vi "Cam.vi"() -> ()   [LabVIEW 2021]
uses:
  <vilib>/userdefined/High Color/IMAQdx.ctl
  <vilib>/MakerHub/LINX/Public/Peripherals/Digital/Digital Write 1 Chan.vi
  <vilib>/MakerHub/LINX/Public/Peripherals/Digital/Digital Write N Chans.vi
  <vilib>/MakerHub/LINX/Private/Local IO/LinxDigitalWrite.vi
  <vilib>/MakerHub/LINX/Public/Utilities/Check Channel.vi
  <vilib>/MakerHub/LINX/Public/Utilities/Open Serial.vi
  <vilib>/MakerHub/LINX/Private/Utilties/Generate Error.vi
  <vilib>/vision/driver/NI_Vision_Acquisition_Software.lvlib
  <vilib>/vision/NI_Vision_Development_Module.lvlib
  <vilib>/MakerHub/LINX/LMH-LINX.lvlib
panel:
  out "Loop Rate (Hz)":u32
  in  "Digital Output Channel":u8=13
  in  "Serial Port":refnum<visa-resource-name>
  out "EJE Y":sgl
  out "EJE X":sgl
  in  "Reconocer":bool
  out "Muestra":T1(plugin-control)
  out "Imagen":T1(plugin-control)
  in  "Camara":T2
  in  "stop":bool
  # "ELECTROMARK VISION ARTIFICIAL"
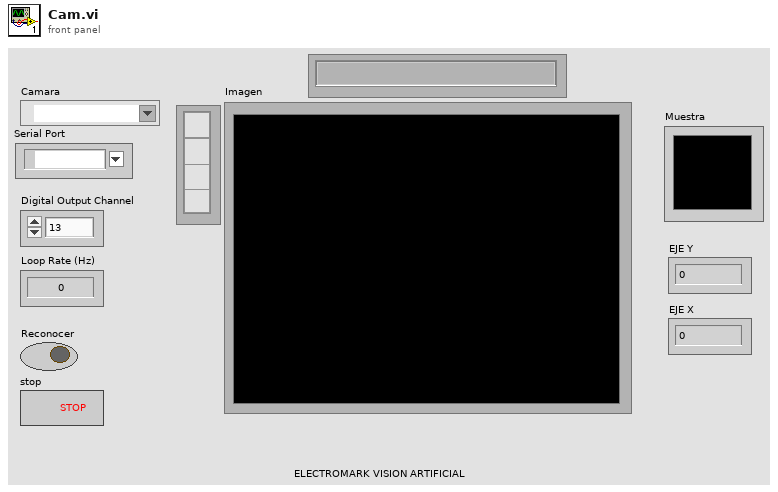
[diagram p1: front panel]
types:
  T1 = typedef "IMAQ Image.ctl" = refnum<image>
  T2 = typedef "IMAQdx.ctl" = refnum<k21>
  T3 = typedef "Image Type" = u32
  T4 = typedef "LMH-LINX.lvlib/LINX Ref.ctl" = cluster{"IO":T5, "Interface":T6, "LINX Device Config":T7}
  T5 = typedef "LMH-LINX.lvlib/Platform.ctl" = enum16{"Remote", "Local"}
  T6 = typedef "LMH-LINX.lvlib/Interface.ctl" = enum16{"Serial", "TCP"}
  T7 = typedef "LMH-LINX.lvlib/Device.lvlib/LINX Device Config.ctl" = cluster{"Interface":T6, "COM Port":refnum<visa-resource-name>, "TCP Configuration":T8, "Device Family":u8, "Device ID":u8, "Device Name":string, "TCP Ref":refnum<k5>, "Channels":T9}
  T8 = typedef "LMH-LINX.lvlib/Device.lvlib/TCP Config.ctl" = cluster{"IP Address":string, "Port":u16}
  T9 = typedef "LMH-LINX.lvlib/Channels.ctl" = cluster{"DI":u8[], "DO":u8[], "AI":u8[], "AO":u8[], "PWM":u8[], "QE":u8[], "UART":u8[], "I2C 2":u8[], "SPI":u8[], "CAN":u8[], "Servo":u8[], "AI Ref (V)":dbl, "AI Resolution (Bits)":u8, "AO Ref (V)":dbl, "AO Resolution (Bits)":u8}
  T10 = cluster{"Match Mode":u16, "Number of Matches Requested":i32, "Minimum Match Score":sgl, "SubPixel Accuracy":bool, "Rotation Angle Ranges":cluster{"Start":sgl, "End":sgl}[], "Show Search Area":bool, "Show Result":bool}
  T11 = cluster{"Position":cluster{"x":sgl, "y":sgl}, "Angle":sgl, "Scale":sgl, "Score":sgl, "Bounding Box":cluster{"x":sgl, "y":sgl}[]}[]
  T12 = cluster{"Matches[0]":cluster{"Position":cluster{"x":sgl, "y":sgl}, "Angle":sgl, "Scale":sgl, "Score":sgl, "Bounding Box":cluster{"x":sgl, "y":sgl}[]}, "Matches[1]":cluster{"Position":cluster{"x":sgl, "y":sgl}, "Angle":sgl, "Scale":sgl, "Score":sgl, "Bounding Box":cluster{"x":sgl, "y":sgl}[]}, "Matches[2]":cluster{"Position":cluster{"x":sgl, "y":sgl}, "Angle":sgl, "Scale":sgl, "Score":sgl, "Bounding Box":cluster{"x":sgl, "y":sgl}[]}, "Matches[3]":cluster{"Position":cluster{"x":sgl, "y":sgl}, "Angle":sgl, "Scale":sgl, "Score":sgl, "Bounding Box":cluster{"x":sgl, "y":sgl}[]}, "Matches[4]":cluster{"Position":cluster{"x":sgl, "y":sgl}, "Angle":sgl, "Scale":sgl, "Score":sgl, "Bounding Box":cluster{"x":sgl, "y":sgl}[]}, "Matches[5]":cluster{"Position":cluster{"x":sgl, "y":sgl}, "Angle":sgl, "Scale":sgl, "Score":sgl, "Bounding Box":cluster{"x":sgl, "y":sgl}[]}, "Matches[6]":cluster{"Position":cluster{"x":sgl, "y":sgl}, "Angle":sgl, "Scale":sgl, "Score":sgl, "Bounding Box":cluster{"x":sgl, "y":sgl}[]}, "Matches[7]":cluster{"Position":cluster{"x":sgl, "y":sgl}, "Angle":sgl, "Scale":sgl, "Score":sgl, "Bounding Box":cluster{"x":sgl, "y":sgl}[]}, "Matches[8]":cluster{"Position":cluster{"x":sgl, "y":sgl}, "Angle":sgl, "Scale":sgl, "Score":sgl, "Bounding Box":cluster{"x":sgl, "y":sgl}[]}}
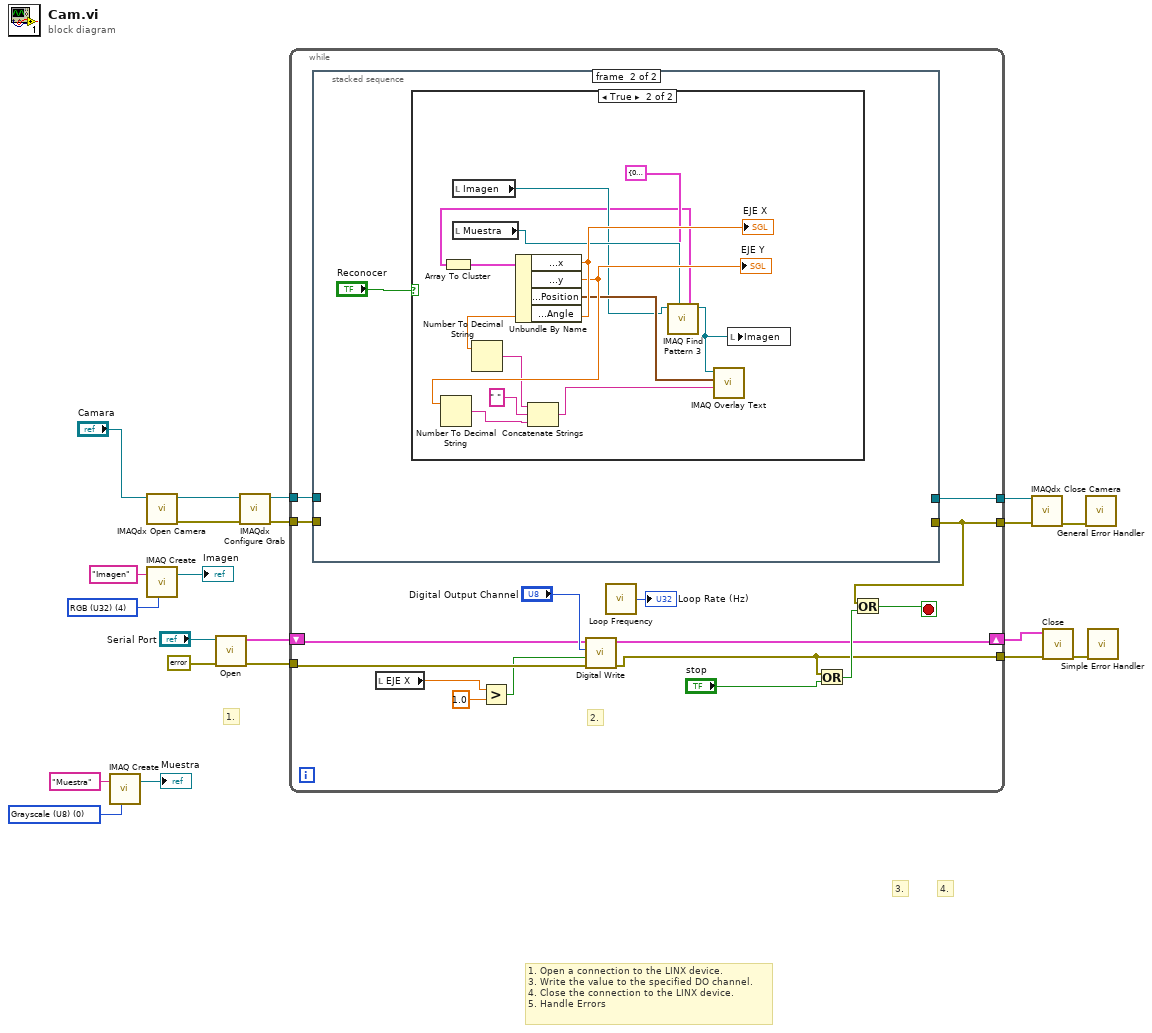
[diagram p0: block diagram]
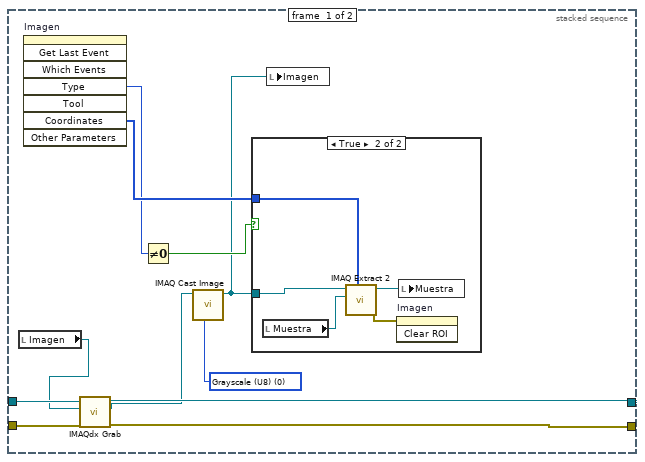
[diagram p2: hidden frame]
diagram:
  w12 = T3 0 items=["Grayscale (U8)", "Grayscale (I16)", "Grayscale (SGL)", "Complex (CSG)", "RGB (U32)", "HSL (U32)", "RGB (U64)", "Grayscale (U16)"] ("Image Type")
  w15 = T3 4 items=["Grayscale (U8)", "Grayscale (I16)", "Grayscale (SGL)", "Complex (CSG)", "RGB (U32)", "HSL (U32)", "RGB (U64)", "Grayscale (U16)"] ("Image Type")
  # "1. Open a connection to the LINX device.\n3. Write the value to the specified DO channel.\n4. Close the connection to the LINX device.\n5. Handle Errors"
  # "4."
  # "3."
  # "1."
  n1 = call "IMAQ Create"("Image Name"="Muestra", "Image Type"=w12) -> ("New Image"=→"Muestra":T1)  [unwired: 3 in, 1 out]
  n2 = call <vilib>:"IMAQdx Open Camera.vi"("Session In"="Camara") -> ("error out"=w19:errorcluster, "Session Out"=w20:T2)  [unwired: 9 in]
  n3 = call "IMAQ Create"("Image Name"="Imagen", "Image Type"=w15) -> ("New Image"=→"Imagen":T1)  [unwired: 3 in, 1 out]
  n4 = call-poly <vilib>:"Open.vi"("Error In"=errorcluster {"status"=FALSE, "code"=0, "source"=""}, "Serial Port"="Serial Port") -> ("Error Out"=w3:errorcluster, "LINX Resource"=w4:T4)  [unwired: 7 in, 1 out]
  n5 = call <vilib>:"IMAQdx Configure Grab.vi"("error in"=w19, "Session In"=w20) -> ("error out"=w18:errorcluster, "Session Out"=w17:T2)  [unwired: 8 in]
  n6 = while {
    tunnel: w18 -> [w37]
    tunnel: w17 -> [w36]
    tunnel: [w35] -> w11
    tunnel: [w33] -> w10
    tunnel: w3 -> [w26]
    tunnel: [w25] -> w1
    shift-right: [w27] -> w2
    shift-left: w4 -> [w28]
    stop <- w34 stop-if-true
    # "2."
    n7 = stacked-sequence {
      tunnel: w37 -> [w48 _]
      tunnel: w36 -> [w47 _]
      tunnel: [w46 _] -> w35
      tunnel: [w45 _] -> w33
      frame #0 {
        w44 = T3 0 items=["Grayscale (U8)", "Grayscale (I16)", "Grayscale (SGL)", "Complex (CSG)", "RGB (U32)", "HSL (U32)", "RGB (U64)", "Grayscale (U16)"] ("Image Type")
        n8 = local read "Imagen"() -> (w41:T1)
        n9 = invoke on="Imagen" class="ImageControl" method="Get Last Event"() -> ("Type"=w39:i32, "Coordinates"=w43:i32[])  [unwired: 8 in, 6 out]
        n10 = call <vilib>:"IMAQdx Grab.vi"("error in"=w48, "Image In"=w41, "Session In"=w47) -> ("error out"=w45:errorcluster, "Image Out"=w38:T1, "Session Out"=w46:T2)  [unwired: 5 in, 1 out]
        n11 = Not Equal To 0?(x=w39) -> (x != 0?=w42:bool)
        n12 = call "IMAQ Cast Image"("Image Type"=w44, "Image Src"=w38) -> ("Image Dst Out"=w40:T1)  [unwired: 8 in, 1 out]
        n13 = case shown="True" w42 {
          tunnel: w40 -> [_ w52]
          tunnel: w43 -> [_ w53]
          frame False {
          }
          frame True {
            n14 = local read "Muestra"() -> (w50:T1)
            n15 = call "IMAQ Extract 2"("Optional Rectangle"=w53, "Image Dst"=w50, "Image Src"=w52) -> ("error out"=w49:errorcluster, "Image Dst Out"=w51:T1)  [unwired: 7 in]
            n16 = invoke on="Imagen" class="ImageControl" method="Clear ROI"(error in=w49) -> ()  [unwired: 2 in, 3 out]
            n17 = local write "Muestra"(w51) -> ()
          }
        }
        n18 = local write "Imagen"(w40) -> ()
      }
      frame #1 {
        n19 = case shown="True" "Reconocer" {
          frame False {
          }
          frame True {
            n20 = local read "Imagen"() -> (w58:T1)
            n21 = local read "Muestra"() -> (w59:T1)
            n22 = call "IMAQ Find Pattern 3"("Settings"=T10 {"Match Mode"=0, "Number of Matches Requested"=1, "Minimum Match Score"=800.0, "SubPixel Accuracy"=FALSE, "Rotation Angle Ranges"=[], "Show Search Area"=TRUE, "Show Result"=TRUE}, "Template"=w59, "Image"=w58) -> ("Image Out"=w56:T1, "Matches"=w55:T11)  [unwired: 3 in, 4 out]
            n23 = Array To Cluster(array=w55) -> (cluster=w67:T12)
            n24 = Unbundle By Name(w67) -> ("Matches[0].Position.x"=w66:sgl, "Matches[0].Position.y"=w65:sgl, "Matches[1].Position"=w63:cluster{"x":sgl, "y":sgl})  [unwired: 1 out]
            "EJE X" <- w66
            "EJE Y" <- w65
            n25 = Number To Decimal String(number=w65) -> (decimal integer string=w61:string)  [unwired: 1 in]
            n26 = Number To Decimal String(number=w66) -> (decimal integer string=w64:string)  [unwired: 1 in]
            n27 = Concatenate Strings(w64, " " ("string"), w61) -> (w62:string)
            n28 = call "IMAQ Overlay Text"("String"=w62, "Origin"=w63, "Image"=w56) -> ()  [unwired: 7 in, 2 out]
            n29 = local write "Imagen"(w56) -> ()
          }
        }
      }
    }
    n30 = local read "EJE X"() -> (w22:sgl)
    n31 = Greater?(x=w22, y=1.0) -> (0:w24:bool)
    n32 = call-poly <vilib>:"Digital Write.vi"("Error In"=w26, "Output Value"=w24, "DO Channel"="Digital Output Channel", "LINX Resource"=w28) -> ("Error Out"=w25:errorcluster, "LINX Resource"=w27:T4)  [unwired: 6 in]
    n33 = call <vilib>:"Loop Frequency.vi"() -> ("Loop Rate (Hz)"=→"Loop Rate (Hz)":u32)
    n34 = Or(x=w25, y="stop") -> (x .or. y?=w32:bool)
    n35 = Or(x=w33, y=w32) -> (x .or. y?=w34:bool)
  }
  n36 = call <vilib>:"IMAQdx Close Camera.vi"("error in"=w10, "Session In"=w11) -> ("error out"=w14:errorcluster)  [unwired: 9 in]
  n37 = call <vilib>:"Close.vi"("Error In"=w1, "LINX Resource"=w2) -> ("Error Out"=w6:errorcluster)  [unwired: 9 in]
  n38 = call <vilib>:"General Error Handler.vi"("error in (no error)"=w14) -> ()  [unwired: 10 in, 5 out]
  n39 = call <vilib>:"Simple Error Handler.vi"("error in (no error)"=w6) -> ()  [unwired: 4 in, 5 out]
